vi "vipmUpdate.vi"() -> (0 "error out":errorcluster)   [LabVIEW 2014, in "lv-cli-steps.lvlib"]
uses:
  lv-cli-steps.lvlib
  <vilib>/Utility/error.llb/DialogType.ctl
  <vilib>/Wiresmith Technology/LabVIEW CLI/CLI Class/CLI.lvclass
  <vilib>/JKI/VIPM API/VIPM API_vipm_api.lvlib
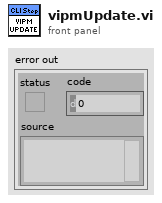
[diagram p1: front panel]
types:
  T1 = typedef "DialogType.ctl" = u16
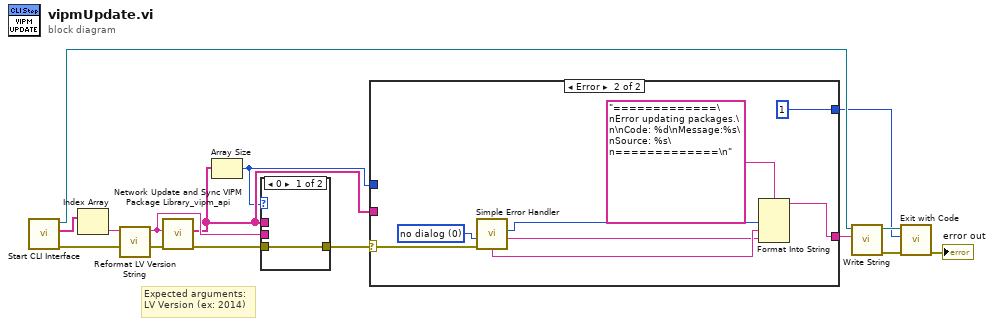
[diagram p0: block diagram]
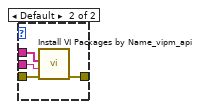
[diagram p2: hidden frame]
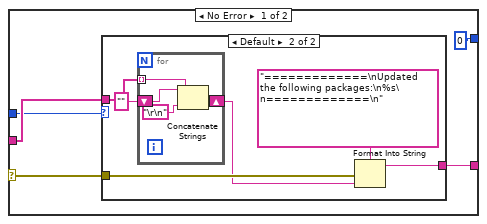
[diagram p3: hidden frame]
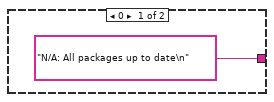
[diagram p4: hidden frame]
diagram:
  # "Expected arguments:\nLV Version (ex: 2014)"
  n1 = call <vilib>:"Start CLI Interface.vi"() -> ("error out"=w5:errorcluster, "Custom Parameters"=w14:string[], "CLI out"=w12:refnum<class "CLI.lvclass">)  [unwired: 9 in]
  n2 = Index Array(array=w14) -> (element=w4:string)  [unwired: 1 in]
  n3 = call "Reformat LV Version String.vi"("Version String (2014)"=w4) -> ("Short Version String (14.0)"=w3:string)  [unwired: 10 in]
  n4 = call <vilib>:"Network Update and Sync VIPM Package Library_vipm_api.vi"("error in (no error)"=w5, "LabVIEW Version"=w3) -> ("error out"=w7:errorcluster, "New Package Updates"=w2:string[])  [unwired: 8 in]
  n5 = Array Size(array=w2) -> (size(s)=w1:i32)
  n6 = case shown="0" w1 {
    tunnel: w7 -> [w15 w19]
    tunnel: [w15 w18] -> w6
    tunnel: w2 -> [_ w17]
    tunnel: w3 -> [_ w16]
    frame 0 {
    }
    frame Default {
      n7 = call <vilib>:"Install VI Packages by Name_vipm_api.vi"("error in (no error)"=w19, "LabVIEW Version"=w16, "Package Names to Install []"=w17) -> ("error out"=w18:errorcluster)  [unwired: 8 in]
    }
  }
  n8 = case shown="Error" w6 {
    selector: w6 -> [w24 w42]
    tunnel: w2 -> [w21 _]
    tunnel: [w23 w43] -> w13
    tunnel: [0 ("Exit Code (0)") 1 ("Exit Code (0)")] -> w9
    tunnel: w1 -> [w20 _]
    frame No Error {
      n9 = case shown="Default" w20 {
        tunnel: w24 -> [_ w30]
        tunnel: ["N/A: All packages up to date\n" w29] -> w23
        tunnel: w21 -> [_ w28]
        frame 0 {
        }
        frame Default {
          n10 = for {
            tunnel: w28 -> [w35] mode=indexing
            shift-right: [w33] -> w26
            shift-left: "" -> [w32]
            n11 = Concatenate Strings(w32, w35, "\r\n") -> (w33:string)
          }
          n12 = Format Into String(format string="=============\nUpdated the following packages:\n%s\n=============\n", error in=w30, w26) -> (resulting string=w29:string)  [unwired: 1 in, 1 out]
        }
      }
    }
    frame Error {
      w41 = T1 0 items=["no dialog", "OK message", "continue or stop message", "OK message + warnings", "continue/stop + warnings"] ("type of dialog (OK msg:1)")
      n13 = call <vilib>:"Simple Error Handler.vi"("type of dialog (OK msg:1)"=w41, "error in (no error)"=w42) -> ("code out"=w38:i32, "source out"=w36:string, "message"=w37:string)  [unwired: 3 in, 2 out]
      n14 = Format Into String(format string="=============\nError updating packages.\n\nCode: %d\nMessage:%s\nSource: %s\n=============\n", w38, w37, w36) -> (resulting string=w43:string)  [unwired: 2 in, 1 out]
    }
  }
  n15 = call <vilib>:"Write String.vi"("Text to Write"=w13, "CLI in"=w12) -> ("error out"=w11:errorcluster, "CLI out"=w10:refnum<class "CLI.lvclass">)  [unwired: 8 in]
  n16 = call <vilib>:"Exit with Code.vi"("error in (no error)"=w11, "Exit Code (0)"=w9, "CLI in"=w10) -> ("error out"=→"error out":errorcluster)  [unwired: 8 in]
